vi "MJG_StageRefFollower_v1.vi"(8 "error in":errorcluster, 9 "Stage PID Cluster":T1={"Stage Z PID"={"Kp"=0.0003, "Kd"=0.01, "Ki"=0.0}, "Stage Y PID"={"Kp"=0.0003, "Kd"=0.01, "Ki"=0.0}, "Stage X PID"={"Kp"=0.0003, "Kd"=0.01, "Ki"=0.0}}, 10 "Stage cmd Posit [mm]":dbl[](array[numeric])=[6.0, 6.0, 6.0], 11 "Refnum In":refnum<k20>) -> (0 "error out":errorcluster, 2 "Stage out Posit [mm]":dbl[](array[numeric])=[12.0, 0.0, 0.0], 3 "Refnum out":refnum<k20>)   [LabVIEW 2016]
uses:
  <vilib>/rvi/interface/nirviReadWriteControl/nirviReadWriteControl.xnode
  <vilib>/rvi/errors/niLvFpgaAdjustHostInterfaceError.vi
  IRISSV2Soft LV2016/IRISS_FPGA_IO_v2.vi
  MJG/Subsystems/GLOBALVARS.vi
  IRISSoft LV2016/FPGA Bitfiles/IRISSControl_FPGATarget_IRISSFPGAIOv2_OF6O1Tw8rps.lvbitx
  <vilib>/rvi/errors/niLvFpgaMergeErrorWithErrorCode.vi
panel:
  # ">>>"
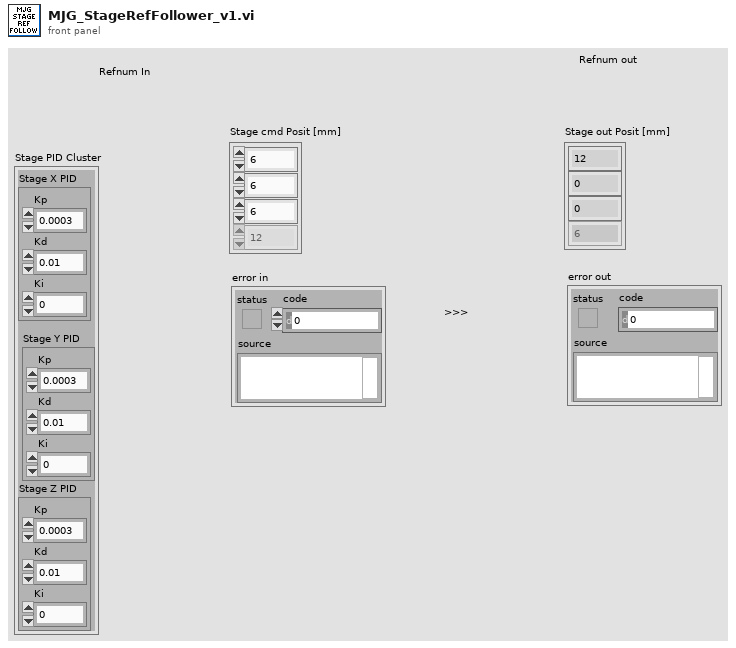
[diagram p1: front panel]
types:
  T1 = cluster{"Stage Z PID":cluster{"Kp":dbl, "Kd":dbl, "Ki":dbl}, "Stage Y PID":cluster{"Kp":dbl, "Kd":dbl, "Ki":dbl}, "Stage X PID":cluster{"Kp":dbl, "Kd":dbl, "Ki":dbl}}
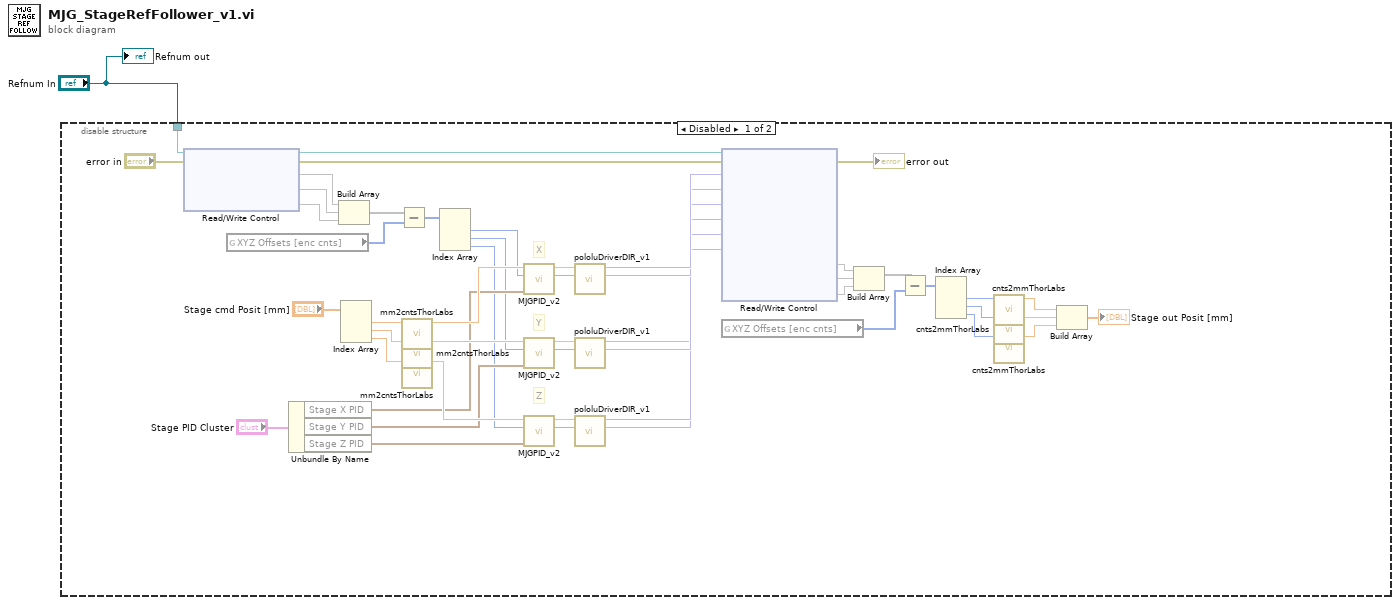
[diagram p0: block diagram]
diagram:
  n1 = disable-structure shown="Disabled" {
    disable-tunnel: "Refnum In" -> [w20 _]
    frame Disabled {
      # "X"
      # "Y"
      # "Z"
      n2 = xnode "Read/Write Control"("FPGA VI Reference In"=w20, "error in"="error in") -> ("FPGA VI Reference Out"=w36:refnum<k20>, "error out"=w35:errorcluster, "X Stage Enc Count"=w16, "Y Stage Enc Count"=w14, "Z Stage Enc Count"=w12)
      n3 = global read "GLOBALVARS.vi" "XYZ Offsets [enc cnts]"() -> (w18:i32[])
      n4 = Unbundle By Name("Stage PID Cluster") -> ("Stage X PID"=w27:cluster{"Kp":dbl, "Kd":dbl, "Ki":dbl}, "Stage Y PID"=w26:cluster{"Kp":dbl, "Kd":dbl, "Ki":dbl}, "Stage Z PID"=w25:cluster{"Kp":dbl, "Kd":dbl, "Ki":dbl})
      n5 = Build Array(w16, w14, w12) -> (w19:void[])
      n6 = Index Array(array="Stage cmd Posit [mm]") -> (element #1=w43:dbl, element #2=w42:dbl, element #3=w41:dbl)  [unwired: 3 in]
      n7 = Subtract(x=w19, y=w18) -> (x-y=w17:i32[])
      n8 = call "mm2cntsThorLabs.vi"("XYX cmd [mm]"=w43) -> ("XYZ cmd [enc cnts]"=w40:dbl)  [unwired: 10 in]
      n9 = call "mm2cntsThorLabs.vi"("XYX cmd [mm]"=w42) -> ("XYZ cmd [enc cnts]"=w39:dbl)  [unwired: 10 in]
      n10 = call "mm2cntsThorLabs.vi"("XYX cmd [mm]"=w41) -> ("XYZ cmd [enc cnts]"=w38:dbl)  [unwired: 10 in]
      n11 = Index Array(array=w17) -> (element #1=w15:i32, element #2=w13:i32, element #3=w11:i32)  [unwired: 3 in]
      n12 = call "MJGPID_v2.vi"("PID Gains"=w27, "Encoder Position"=w15, "Reference"=w40) -> ("Direction"=w33:bool, "Duty Cycle"=w34:dbl)  [unwired: 7 in]
      n13 = call "MJGPID_v2.vi"("PID Gains"=w26, "Encoder Position"=w13, "Reference"=w39) -> ("Direction"=w31:bool, "Duty Cycle"=w32:dbl)  [unwired: 7 in]
      n14 = call "MJGPID_v2.vi"("PID Gains"=w25, "Encoder Position"=w11, "Reference"=w38) -> ("Direction"=w29:bool, "Duty Cycle"=w30:dbl)  [unwired: 7 in]
      n15 = call "pololuDriverDIR_v1.vi"("Direction"=w33, "Duty Cycle"=w34) -> ("PWM 2 Out"=w49:fxp<+,32,0>, "PWM 1 Out"=w50:fxp<+,32,0>)  [unwired: 8 in]
      n16 = call "pololuDriverDIR_v1.vi"("Direction"=w31, "Duty Cycle"=w32) -> ("PWM 2 Out"=w48:fxp<+,32,0>, "PWM 1 Out"=w47:fxp<+,32,0>)  [unwired: 8 in]
      n17 = call "pololuDriverDIR_v1.vi"("Direction"=w29, "Duty Cycle"=w30) -> ("PWM 2 Out"=w45:fxp<+,32,0>, "PWM 1 Out"=w46:fxp<+,32,0>)  [unwired: 8 in]
      n18 = xnode "Read/Write Control"("FPGA VI Reference In"=w36, "error in"=w35, "X PWM 1"=w50, "X PWM 2"=w49, "Y PWM 1"=w47, "Y PWM 2"=w48, "Z PWM 1"=w46, "Z PWM 2"=w45) -> ("error out"=→"error out":errorcluster, "X Stage Enc Count"=w10, "Y Stage Enc Count"=w9, "Z Stage Enc Count"=w8)  [unwired: 1 out]
      n19 = global read "GLOBALVARS.vi" "XYZ Offsets [enc cnts]"() -> (w6:i32[])
      n20 = Build Array(w10, w9, w8) -> (w7:void[])
      n21 = Subtract(x=w7, y=w6) -> (x-y=w5:i32[])
      n22 = Index Array(array=w5) -> (element #1=w4:i32, element #2=w3:i32, element #3=w2:i32)  [unwired: 3 in]
      n23 = call "cnts2mmThorLabs.vi"("XYX cmd [enc cnts]"=w4) -> ("XYZ cmd [mm]"=w24:dbl)  [unwired: 10 in]
      n24 = call "cnts2mmThorLabs.vi"("XYX cmd [enc cnts]"=w3) -> ("XYZ cmd [mm]"=w23:dbl)  [unwired: 10 in]
      n25 = call "cnts2mmThorLabs.vi"("XYX cmd [enc cnts]"=w2) -> ("XYZ cmd [mm]"=w22:dbl)  [unwired: 10 in]
      n26 = Build Array(w24, w23, w22) -> (→"Stage out Posit [mm]":dbl[])
    }
    frame Enabled {
    }
  }
  "Refnum out" <- "Refnum In"
